vi "Test7.vi"() -> ()   [LabVIEW 2010]
uses:
  <vilib>/MDSplus/Library/MDSplus.lvlib
panel:
  in  "SGL array in":sgl[](array[numeric])=[1.11, 2.22, 3.33, 4.44]
  out "SGL out 2":sgl
  out "SGL out":sgl
  out "SGL array out":sgl[](array[numeric])
  in  "Value":sgl=6.666
  in  "Path":string=":NUMX"
  in  "Mode":string="EDIT"
  in  "Shot":i32=-1
  in  "Name":string="my_tree"
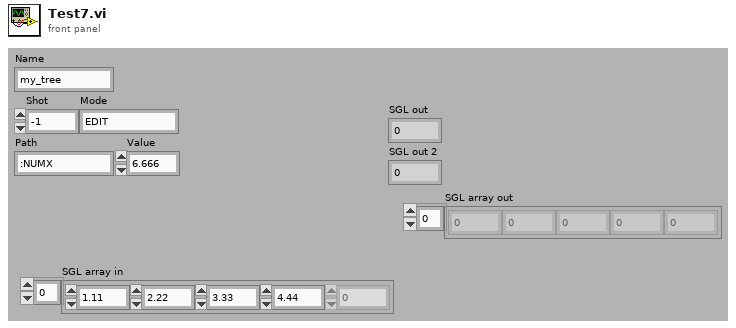
[diagram p1: front panel]
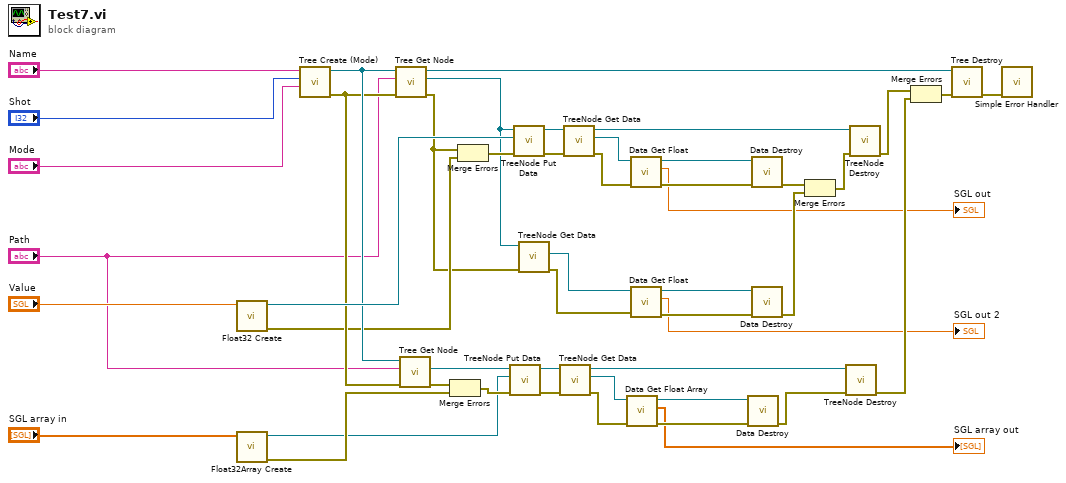
[diagram p0: block diagram]
diagram:
  n1 = call <vilib>:"Float32 Create.vi"("SGL in"="Value") -> ("error out"=w24:errorcluster, "Float32 DVR out"=w38:refnum<data-value>)  [unwired: 9 in]
  n2 = call <vilib>:"Float32Array Create.vi"("SGL array in"="SGL array in") -> ("error out"=w22:errorcluster, "Float32Array DVR out"=w9:refnum<data-value>)  [unwired: 9 in]
  n3 = call <vilib>:"Tree Create (Mode).vi"("Mode"="Mode", "Shot"="Shot", "Name"="Name") -> ("error out"=w26:errorcluster, "Tree DVR out"=w27:refnum<data-value>)  [unwired: 7 in]
  n4 = call <vilib>:"Tree Get Node.vi"("error in (no error)"=w26, "Path"="Path", "Tree DVR in"=w27) -> ("error out"=w13:errorcluster, "Node out"=w14:refnum<data-value>, "Tree DVR out"=w39:refnum<data-value>)  [unwired: 6 in]
  n5 = call <vilib>:"Tree Get Node.vi"("error in (no error)"=w26, "Path"="Path", "Tree DVR in"=w27) -> ("error out"=w21:errorcluster, "Node out"=w25:refnum<data-value>)  [unwired: 6 in, 1 out]
  n6 = Merge Errors(w21, w22) -> (w20:errorcluster)
  n7 = Merge Errors(w13, w24) -> (w23:errorcluster)
  n8 = call <vilib>:"TreeNode Put Data.vi"("error in (no error)"=w20, "Data"=w9, "TreeNode DVR in"=w25) -> ("error out"=w34:errorcluster, "TreeNode DVR out"=w33:refnum<data-value>)  [unwired: 7 in]
  n9 = call <vilib>:"TreeNode Put Data.vi"("error in (no error)"=w23, "Data"=w38, "TreeNode DVR in"=w14) -> ("error out"=w35:errorcluster, "TreeNode DVR out"=w36:refnum<data-value>)  [unwired: 7 in]
  n10 = call <vilib>:"TreeNode Get Data.vi"("error in (no error)"=w13, "TreeNode DVR in"=w14) -> ("error out"=w5:errorcluster, "Data out"=w4:refnum<data-value>)  [unwired: 7 in, 1 out]
  n11 = call <vilib>:"TreeNode Get Data.vi"("error in (no error)"=w34, "TreeNode DVR in"=w33) -> ("error out"=w28:errorcluster, "Data out"=w6:refnum<data-value>, "TreeNode DVR out"=w31:refnum<data-value>)  [unwired: 7 in]
  n12 = call <vilib>:"TreeNode Get Data.vi"("error in (no error)"=w35, "TreeNode DVR in"=w36) -> ("error out"=w43:errorcluster, "Data out"=w44:refnum<data-value>, "TreeNode DVR out"=w40:refnum<data-value>)  [unwired: 7 in]
  n13 = call <vilib>:"Data Get Float Array.vi"("error in (no error)"=w28, "Data DVR in"=w6) -> ("error out"=w30:errorcluster, "SGL array out"=→"SGL array out":sgl[], "Data DVR out"=w29:refnum<data-value>)  [unwired: 6 in, 1 out]
  n14 = call <vilib>:"Data Get Float.vi"("error in (no error)"=w43, "Data DVR in"=w44) -> ("error out"=w41:errorcluster, "SGL out"=→"SGL out":sgl, "Data DVR out"=w42:refnum<data-value>)  [unwired: 7 in]
  n15 = call <vilib>:"Data Get Float.vi"("error in (no error)"=w5, "Data DVR in"=w4) -> ("error out"=w15:errorcluster, "SGL out"=→"SGL out 2":sgl, "Data DVR out"=w16:refnum<data-value>)  [unwired: 7 in]
  n16 = call <vilib>:"Data Destroy.vi"("error in (no error)"=w30, "Data DVR in"=w29) -> ("error out"=w32:errorcluster)  [unwired: 9 in]
  n17 = call <vilib>:"Data Destroy.vi"("error in (no error)"=w41, "Data DVR in"=w42) -> ("error out"=w11:errorcluster)  [unwired: 9 in]
  n18 = call <vilib>:"Data Destroy.vi"("error in (no error)"=w15, "Data DVR in"=w16) -> ("error out"=w12:errorcluster)  [unwired: 9 in]
  n19 = Merge Errors(w11, w12) -> (w10:errorcluster)
  n20 = call <vilib>:"TreeNode Destroy.vi"("error in (no error)"=w32, "TreeNode DVR in"=w31) -> ("error out"=w19:errorcluster)  [unwired: 9 in]
  n21 = call <vilib>:"TreeNode Destroy.vi"("error in (no error)"=w10, "TreeNode DVR in"=w40) -> ("error out"=w18:errorcluster)  [unwired: 9 in]
  n22 = Merge Errors(w18, w19) -> (w17:errorcluster)
  n23 = call <vilib>:"Tree Destroy.vi"("error in (no error)"=w17, "Tree DVR in"=w39) -> ("error out"=w37:errorcluster)  [unwired: 9 in]
  n24 = call <vilib>:"Simple Error Handler.vi"("error in (no error)"=w37) -> ()  [unwired: 4 in, 5 out]
